vi "Notifier get and set.vi"(6 "Operation":enum16{"Init", "Get", "Set"}(ring)=enum."Get", 8 "error in":errorcluster, 10 "notifier In":refnum<notifier>) -> (0 "error out":errorcluster, 2 "notifier out":refnum<notifier>)   [LabVIEW 2021]
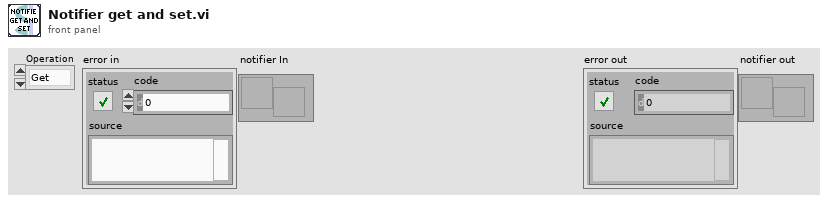
[diagram p1: front panel]
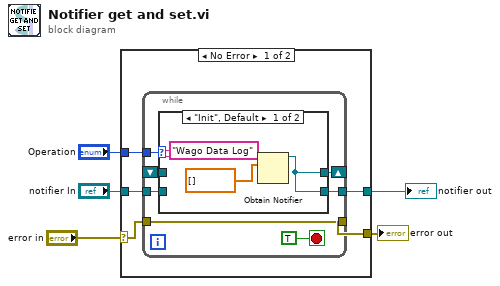
[diagram p0: block diagram]
diagram:
  n1 = case shown="No Error" "error in" {
    selector: "error in" -> [w7 w23]
    tunnel: "Operation" -> [w10 _]
    tunnel: "notifier In" -> [w9 w22]
    tunnel: [w8 w22] -> w3
    tunnel: [w6 w23] -> w1
    frame No Error {
      n2 = while {
        tunnel: w10 -> [w16]
        tunnel: w9 -> [w15]
        shift-right: [w14] -> _
        shift-left: _ -> [w12]
        tunnel: [w13] -> w8
        tunnel: w7 -> [w11]
        tunnel: [w11] -> w6
        stop <- TRUE stop-if-true
        n3 = case shown="\"Init\", Default" w16 {
          tunnel: w15 -> [_ _]
          tunnel: [w18 w21] -> w14
          tunnel: [w18 w21] -> w13
          tunnel: w12 -> [_ w21]
          frame "Init", Default {
            n4 = Obtain Notifier(name (unnamed)="Wago Data Log", notification data type=dbl[] [] ("initialized array")) -> (notifier out=w18:refnum<notifier>)  [unwired: 2 in, 2 out]
          }
          frame "Get" {
          }
        }
      }
    }
    frame Error {
    }
  }
  "error out" <- w1
  "notifier out" <- w3
